vi "DemoMaybe.vi"() -> ()   [LabVIEW 2019, in "C4209 PNA.lvclass"]
uses:
  C4209 PNA.lvclass
  N5222A PNA/N5222AConfig.ctl
panel:
  out "error out":errorcluster
  out "text":string
  in  "C4209 Cfg":T1={"ResourceName"="", "Enable"=FALSE, "Channel"=1, "CalFileName"="", "MeasName"="", "TempDatFile"="", "Power, dBm"=-30.0, "NumPoints"=201, "Start Freq, Hz"=5000000000.0, "Stop Freq, Hz"=6000000000.0, "NumAverages"=20, "Sweep Type"=0, "IF Bandwidth"=0.0} {"Sweep Type" items=["Linear Frequency", "Log Frequency", "Power Sweep", "CW Time"]; "Stop Freq, Hz" format="%_3p"; "Start Freq, Hz" format="%_3p"}
  in  "error in (no error)":errorcluster
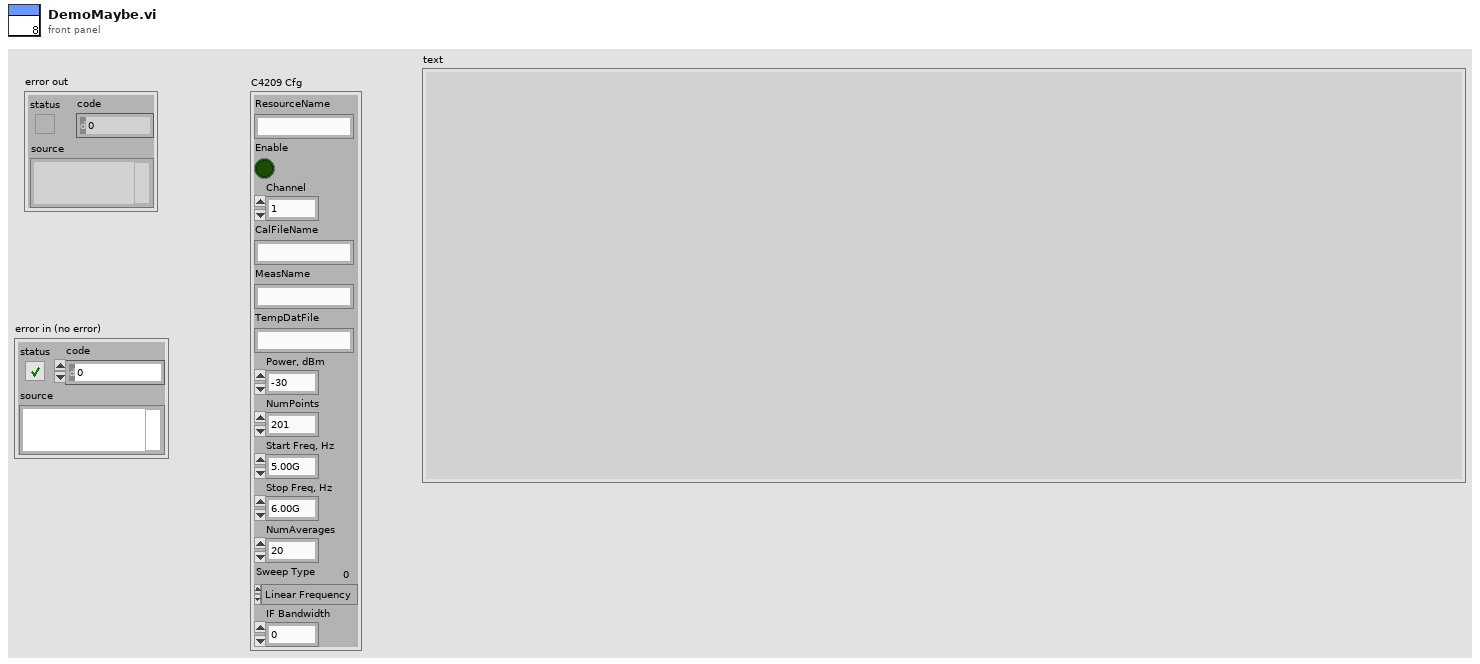
[diagram p1: front panel]
types:
  T1 = typedef "N5222AConfig.ctl" = cluster{"ResourceName":string, "Enable":bool, "Channel":i32, "CalFileName":string, "MeasName":string, "TempDatFile":string, "Power, dBm":dbl, "NumPoints":i32, "Start Freq, Hz":dbl, "Stop Freq, Hz":dbl, "NumAverages":i32, "Sweep Type":i32, "IF Bandwidth":dbl}
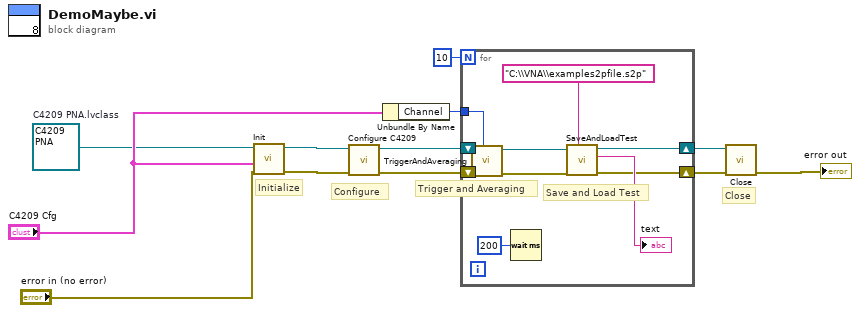
[diagram p0: block diagram]
diagram:
  w2 = refnum<class "C4209 PNA.lvclass"> refnum  # C4209 PNA.lvclass
  # "Close"
  # "Configure"
  # "Initialize"
  n1 = call "Init.vi"("error in (no error)"="error in (no error)", "C4209 Cfg"="C4209 Cfg", "C4209 PNA"=w2) -> ("error out"=w10:errorcluster, "C4209 PNA out"=w11:refnum<class "C4209 PNA.lvclass">)  [unwired: 7 in]
  n2 = call "Configure C4209.vi"("error in (no error)"=w10, "C4209 PNA"=w11) -> ("error out"=w8:errorcluster, "C4209 PNA out"=w9:refnum<class "C4209 PNA.lvclass">)  [unwired: 8 in]
  n3 = Unbundle By Name("C4209 Cfg") -> ("Channel"=w7:i32)
  n4 = for {
    N: 10 -> [_]
    tunnel: w7 -> [w20]
    shift-right: [w14] -> w4
    shift-left: w9 -> [w22]
    shift-right: [w15] -> w5
    shift-left: w8 -> [w21]
    # "Save and Load Test"
    # "Trigger and Averaging"
    n5 = call "TriggerAndAveraging.vi"("Channel"=w20, "error in (no error)"=w21, "C4209 PNA"=w22) -> ("error out"=w18:errorcluster, "C4209 PNA out"=w19:refnum<class "C4209 PNA.lvclass">)  [unwired: 7 in]
    n6 = Wait (ms)(milliseconds to wait=u32 200) -> ()  [unwired: 1 out]
    n7 = call "SaveAndLoadTest.vi"("File Name ()"="C:\\VNA\\examples2pfile.s2p", "error in (no error)"=w18, "C4209 PNA"=w19) -> ("error out"=w15:errorcluster, "text"=→"text":string, "C4209 PNA out"=w14:refnum<class "C4209 PNA.lvclass">)  [unwired: 6 in]
  }
  n8 = call "Close.vi"("error in (no error)"=w5, "C4209 PNA"=w4) -> ("error out"=→"error out":errorcluster)  [unwired: 8 in, 1 out]
